vi "Control Sain Board Relays.vi"(0 "Mode":T1, 5 "error in":errorcluster, 6 "Device Name":string="Dev1") -> (19 "error out":errorcluster)   [LabVIEW 2015]
uses:
  Sain Relays Mode.ctl
  <vilib>/DAQmx/write.llb/DAQmx Write (Digital 1D Bool 1Chan 1Samp).vi
  <vilib>/DAQmx/create/channels.llb/DAQmx Create Channel (DO-Digital Output).vi
  <vilib>/DAQmx/miscellaneous.llb/DAQmx Fill In Error Info.vi
panel:
  out "Array":bool[](array[boolean])=[TRUE, TRUE, TRUE, FALSE, TRUE, TRUE, TRUE, TRUE, FALSE, FALSE, FALSE, FALSE, FALSE, FALSE, TRUE, FALSE]
  # "K1 Not Used\nK2 Not Used\nK3 Not Used\n---->K4 Interlock\nK5 Not Used\nK6 Not Used\nK7 Not Used\nK8 Not Used\nK9 REF-2.5\nK10 +3.3V\nK11 +5.2V\nK12 +5.2VA\nK13 -5.2VA\nK14 +1.6V\nK15  unused\n---->K16   VBAT"
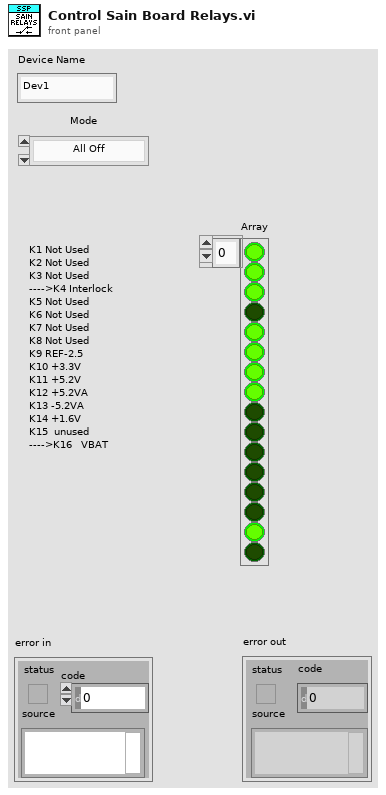
[diagram p1: front panel]
types:
  T1 = typedef "Sain Relays Mode.ctl" = enum16{"All Off", "Enable"}
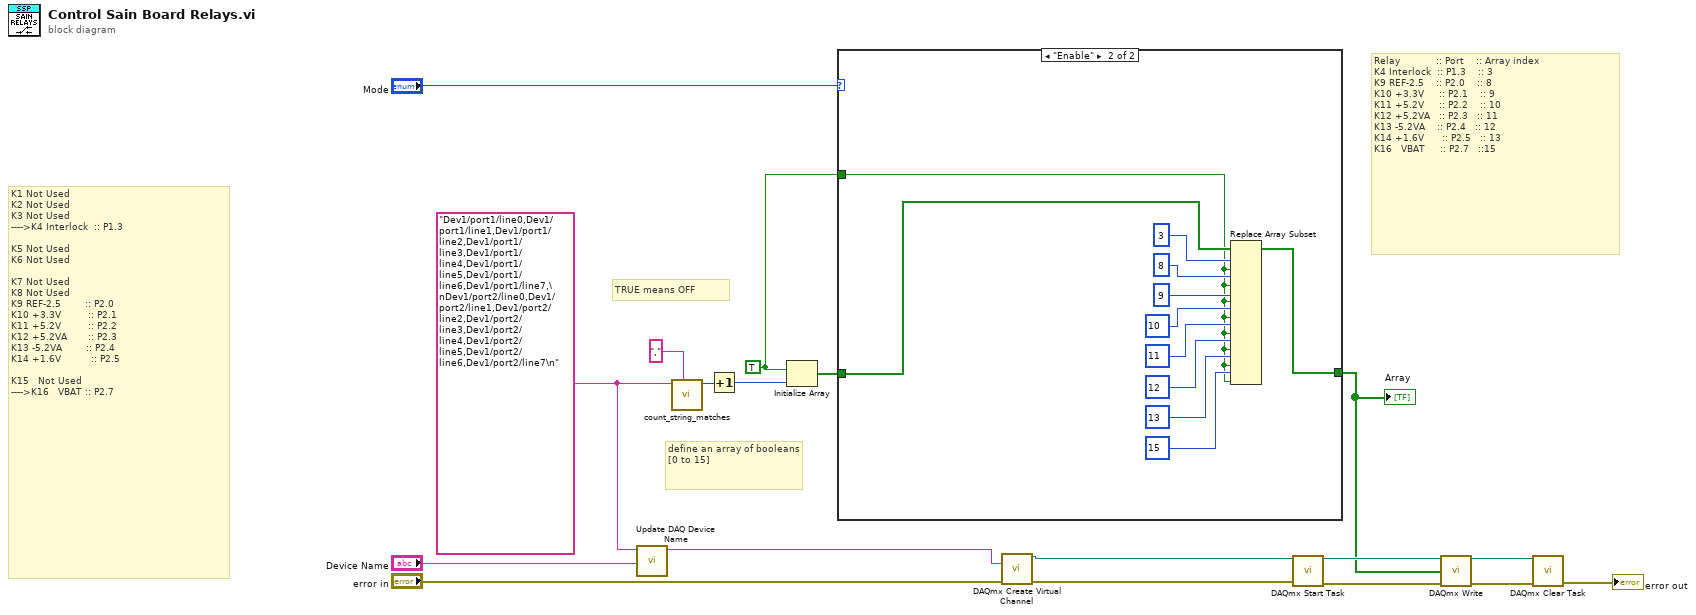
[diagram p0: block diagram]
diagram:
  w4 = "Dev1/port1/line0,Dev1/port1/line1,Dev1/port1/line2,Dev1/port1/line3,Dev1/port1/line4,Dev1/port1/line5,Dev1/port1/line6,Dev1/port1/line7,\nDev1/port2/line0,Dev1/port2/line1,Dev1/port2/line2,Dev1/port2/line3,Dev1/port2/line4,Dev1/port2/line5,Dev1/port2/line6,Dev1/port2/line7\n"
  w3 = TRUE
  # "define an array of booleans [0 to 15]"
  # "Relay            :: Port    :: Array index\nK4 Interlock  :: P1.3    :: 3\nK9 REF-2.5    :: P2.0    :: 8\nK10 +3.3V     :: P2.1    :: 9\nK11 +5.2V     :: P2.2    :: 10\nK12 +5.2VA   :: P2.3   :: 11\nK13 -5.2VA    :: P2.4   :: 12\nK14 +1.6V      :: P2.5   :: 13\nK16   VBAT     :: P2.7   ::15"
  # "K1 Not Used\nK2 Not Used\nK3 Not Used\n---->K4 Interlock  :: P1.3\n\nK5 Not Used\nK6 Not Used\n\nK7 Not Used\nK8 Not Used\nK9 REF-2.5        :: P2.0\nK10 +3.3V         :: P2.1\nK11 +5.2V         :: P2.2\nK12 +5.2VA       :: P2.3\nK13 -5.2VA        :: P2.4\nK14 +1.6V          :: P2.5\n\nK15   Not Used\n---->K16   VBAT :: P2.7"
  # "TRUE means OFF"
  n1 = call "Update DAQ Device Name.vi"("Device Name"="Device Name", "Lines in (String)"=w4) -> ("Lines out (DAQmx Physical Channels)"=w7:tag)  [unwired: 9 in]
  n2 = call "count_string_matches.vi"("String"=w4, "String to Match"=",") -> ("Number of matches"=w6:i32)  [unwired: 7 in, 1 out]
  n3 = Increment(x=w6) -> (x+1=w2:i32)
  n4 = Initialize Array(w3, w2) -> (w1:bool[])
  n5 = case shown="\"Enable\"" "Mode" {
    tunnel: w3 -> [_ w20]
    tunnel: [w19 w30] -> w8
    tunnel: w1 -> [w19 w21]
    frame "All Off", Default {
    }
    frame "Enable" {
      n6 = Replace Array Subset(array=w21, new element #1=w20, index #1=3 ("index"), new element #2=w20, index #2=8 ("index"), new element #3=w20, index #3=9 ("index"), new element #4=w20, index #4=10 ("index"), new element #5=w20, index #5=11 ("index"), new element #6=w20, index #6=12 ("index"), new element #7=w20, index #7=13 ("index"), new element #8=w20, index #8=15 ("index")) -> (w30:bool[])
    }
  }
  "Array" <- w8
  n7 = call-poly <vilib>:"DAQmx Create Virtual Channel.vi"("lines"=w7, "error in"="error in") -> ("task out"=w12:refnum<k21>, "error out"=w11:errorcluster)  [unwired: 12 in]
  n8 = call <vilib>:"DAQmx Start Task.vi"("task/channels in"=w12, "error in"=w11) -> ("task out"=w13:refnum<k21>, "error out"=w14:errorcluster)  [unwired: 12 in]
  n9 = call-poly <vilib>:"DAQmx Write.vi"("task/channels in"=w13, "data"=w8, "error in"=w14) -> ("task out"=w15:refnum<k21>, "error out"=w16:errorcluster)  [unwired: 10 in, 1 out]
  n10 = call <vilib>:"DAQmx Clear Task.vi"("task in"=w15, "error in"=w16) -> ("error out"=→"error out":errorcluster)  [unwired: 13 in]
